vi "Find all vi paths in current project.vi"(4 "error in":errorcluster, 7 "ExcludeDependencies?":bool) -> (0 "error out":errorcluster, 2 "Project name":string, 3 "All VIs in .proj":string[](array[string]))   [LabVIEW 2013]
doc: "This .vi returns references to all the .vi's under the My Computer section of the current project This requires that only one project is open. \n\nIf multiple projects are open, he current project has to have the conditional disable symbol : ProjectName with the project name present, and the subdiagram filled out in the subvi."
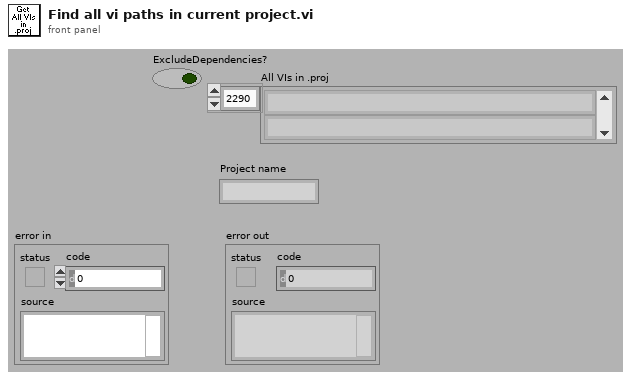
[diagram p1: front panel]
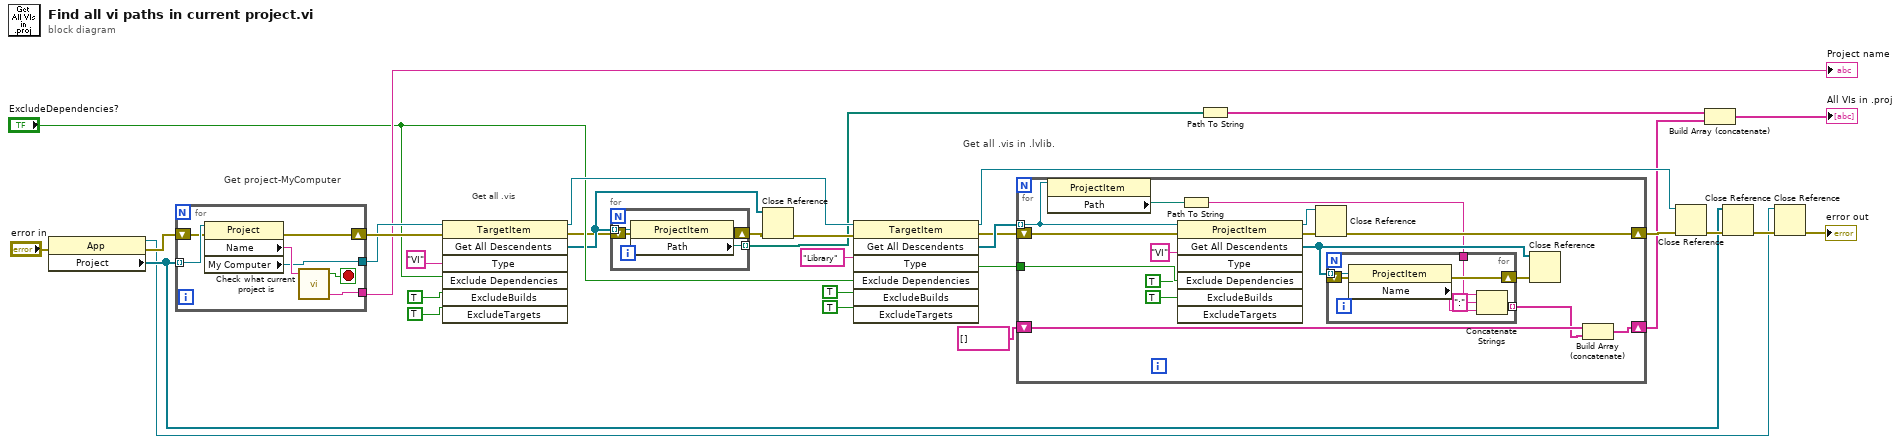
[diagram p0: block diagram]
diagram:
  # "Get project-MyComputer"
  # "Get all .vis in .lvlib."
  # "Get all .vis"
  n1 = property class="App"(error in="error in") -> (reference out=w20:refnum<vi>, error out=w27:errorcluster, "Project"=w22:refnum<vi>[])  [unwired: 1 in]
  n2 = for {
    tunnel: w22 -> [w37] mode=indexing
    shift-right: [w34] -> w30
    shift-left: w27 -> [w35]
    tunnel: [w33] -> w28
    tunnel: [w32] -> w29
    stop <- w38 stop-if-true
    n3 = property class="Project"(reference=w37, error in=w35) -> (error out=w34:errorcluster, "Name"=w36:string, "My Computer"=w32:refnum<vi>)  [unwired: 1 out]
    n4 = call "Check what current project is.vi"("Project Name"=w36) -> ("Project"=w33:string, "Input = Current Project,\nor project not defined?"=w38:bool)  [unwired: 3 out]
  }
  "Project name" <- w28
  n5 = invoke class="TargetItem" method="Get All Descendents"(reference=w29, error in=w30, "Type"="VI", "Exclude Dependencies"="ExcludeDependencies?", "ExcludeBuilds"=TRUE, "ExcludeTargets"=TRUE ("ExcludeBuilds")) -> (reference out=w18:refnum<vi>, error out=w5:errorcluster, "All Descendents"=w6:refnum<vi>[])  [unwired: 1 in, 4 out]
  n6 = for {
    tunnel: w6 -> [w42] mode=indexing
    tunnel: [w41] -> w2 mode=indexing
    shift-right: [w40] -> w7
    shift-left: w5 -> [w39]
    n7 = property class="ProjectItem"(reference=w42, error in=w39) -> (error out=w40:errorcluster, "Path"=w41:path)  [unwired: 1 out]
  }
  n8 = Close Reference(reference=w6, error in (no error)=w7) -> (error out=w4:errorcluster)
  n9 = invoke class="TargetItem" method="Get All Descendents"(reference=w18, error in=w4, "Type"="Library", "Exclude Dependencies"="ExcludeDependencies?", "ExcludeBuilds"=TRUE, "ExcludeTargets"=TRUE) -> (reference out=w17:refnum<vi>, error out=w11:errorcluster, "All Descendents"=w13:refnum<vi>[])  [unwired: 1 in, 4 out]
  n10 = for {
    tunnel: w13 -> [w45] mode=indexing
    tunnel: "ExcludeDependencies?" -> [w57]
    shift-right: [w51] -> w10
    shift-left: w11 -> [w52]
    shift-right: [w49] -> w3
    shift-left: string[] [] -> [w50]
    n11 = property class="ProjectItem"(reference=w45) -> ("Path"=w44:path)  [unwired: 1 in, 2 out]
    n12 = invoke class="ProjectItem" method="Get All Descendents"(reference=w45, error in=w52, "Type"="VI", "Exclude Dependencies"=w57, "ExcludeBuilds"=TRUE, "ExcludeTargets"=TRUE) -> (reference out=w53:refnum<vi>, error out=w54:errorcluster, "All Descendents"=w48:refnum<vi>[])  [unwired: 1 in, 4 out]
    n13 = Path To String(path=w44) -> (string=w43:string)
    n14 = Close Reference(reference=w53, error in (no error)=w54) -> (error out=w51:errorcluster)
    n15 = for {
      tunnel: w48 -> [w65] mode=indexing
      shift-right: [w64] -> w47
      shift-left: _ -> [w63]
      tunnel: [w61] -> w46 mode=indexing
      tunnel: w43 -> [w60]
      n16 = property class="ProjectItem"(reference=w65, error in=w63) -> (error out=w64:errorcluster, "Name"=w62:string)  [unwired: 1 out]
      n17 = Concatenate Strings(w60, ":" ("string"), w62) -> (w61:string)
    }
    n18 = Close Reference(reference=w48, error in (no error)=w47) -> ()  [unwired: 1 out]
    n19 = Build Array (concatenate)(w50, w46) -> (w49:string[])
  }
  n20 = Path To String(path=w2) -> (string=w1:string[])
  n21 = Close Reference(reference=w17, error in (no error)=w10) -> (error out=w23:errorcluster)
  n22 = Build Array (concatenate)(w1, w3) -> (→"All VIs in .proj":string[])
  n23 = Close Reference(reference=w22, error in (no error)=w23) -> (error out=w21:errorcluster)
  n24 = Close Reference(reference=w20, error in (no error)=w21) -> (error out=→"error out":errorcluster)
